vi "hysteresis.vi"(7 "max_inc":dbl, 8 "analog_s":dbl[](array[numeric]), 11 "analog_d":dbl[](array[numeric])) -> (4 "hysteresis?":bool, 5 "max difference a":dbl)   [LabVIEW 2021]
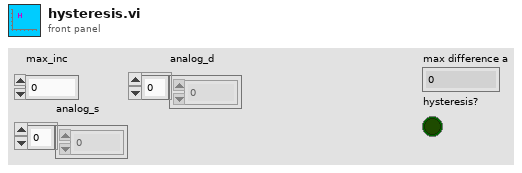
[diagram p1: front panel]
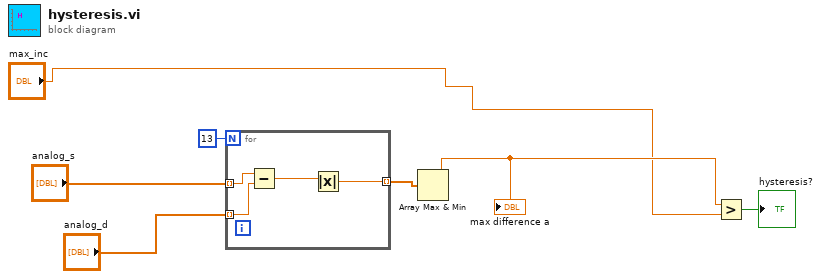
[diagram p0: block diagram]
diagram:
  n1 = for {
    N: 13 -> [_]
    tunnel: "analog_s" -> [w11] mode=indexing
    tunnel: [w9] -> w6 mode=indexing
    tunnel: "analog_d" -> [w8] mode=indexing
    n2 = Subtract(x=w11, y=w8) -> (x-y=w10:dbl)
    n3 = Absolute Value(x=w10) -> (abs(x)=w9:dbl)
  }
  n4 = Array Max & Min(array=w6) -> (max value=w5:dbl)  [unwired: 3 out]
  "max difference a" <- w5
  n5 = Greater?(x=w5, y="max_inc") -> (0:→"hysteresis?":bool)
